vi "启动.vi"() -> ()   [LabVIEW 2016]
uses:
  <vilib>/NI/Progress Bar/Controls/Update Bar Actions.ctl
  <vilib>/NI/Progress Bar/Controls/Progress Bar Properties.ctl
  <vilib>/NI/Progress Bar/Progress Bar.lvlib
panel:
  out "exists?":bool
  out "error out":errorcluster
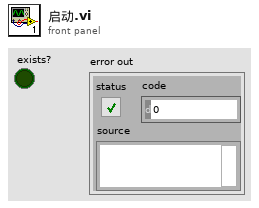
[diagram p1: front panel]
types:
  T1 = enum32{"Invalid", "Standard", "Closed", "Hidden", "Minimized", "Maximized"}
  T2 = typedef "Progress Bar.lvlib/Progress Bar Properties.ctl" = cluster{"Background Color":u32, "Installer Title":string, "Title Color":u32, "Action Text":string, "Text Color":u32, "Slider Value":u8, "Bar Color":u32, "Timeout":i32}
  T3 = typedef "Progress Bar.lvlib/Update Bar Actions.ctl" = enum16{"Add To Existing", "Set to Value"}
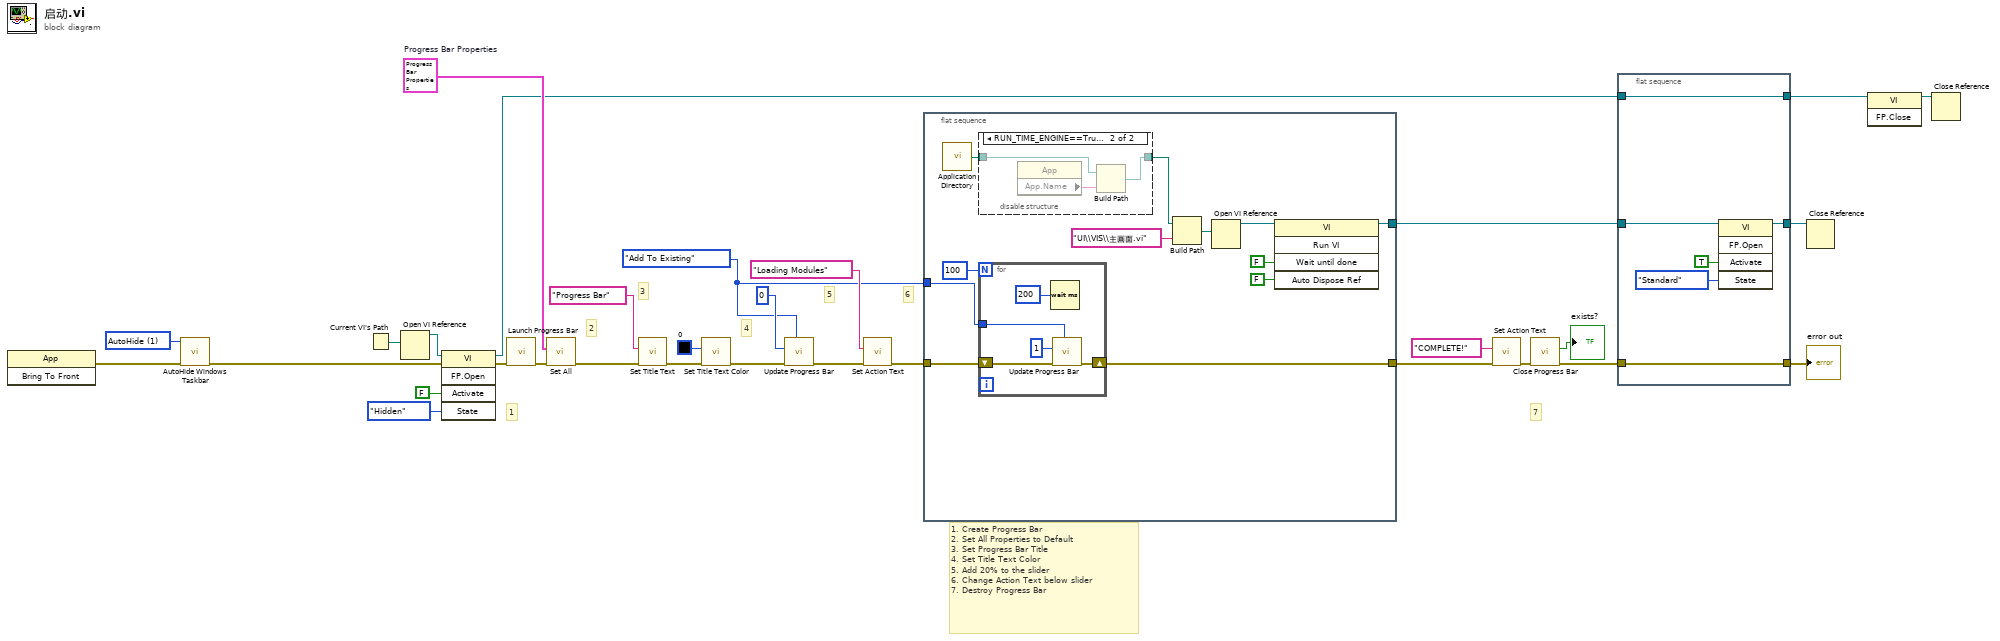
[diagram p0: block diagram]
diagram:
  w4 = u8 1 items=["AutoHide"=1, "AlwaysOnTop"=2] ("Operation")
  w20 = T2 {"Background Color"=3381759, "Installer Title"="Progress", "Title Color"=0, "Action Text"="", "Text Color"=0, "Slider Value"=0, "Bar Color"=6618880, "Timeout"=10000}  # Progress Bar Properties
  w19 = Update_Bar_Actions."Add To Existing" ("Action")
  # "7"
  # "6"
  # "5"
  # "4"
  # "3"
  # "2"
  # "1"
  # "1. Create Progress Bar\n2. Set All Properties to Default\n3. Set Progress Bar Title\n4. Set Title Text Color\n5. Add 20% to the slider\n6. Change Action Text below slider\n7. Destroy Progress Bar"
  n1 = invoke class="App" method="Bring To Front"() -> (error out=w2:errorcluster)  [unwired: 3 in, 2 out]
  n2 = call "AutoHide Windows Taskbar.vi"("error in (no error)"=w2, "Operation"=w4) -> ("error out"=w5:errorcluster)  [unwired: 5 in]
  n3 = Current VI's Path() -> (path=w14:path)
  n4 = Open VI Reference(vi path=w14) -> (vi reference=w15:refnum<vi>)  [unwired: 5 in, 1 out]
  n5 = invoke class="VI" method="FP.Open"(reference=w15, error in=w5, "Activate"=FALSE ("激活？"), "State"=T1."Hidden" ("状态")) -> (reference out=w10:refnum<vi>, error out=w11:errorcluster)  [unwired: 1 in, 3 out]
  n6 = call <vilib>:"Launch Progress Bar.vi"("error in (no error)"=w11) -> ("error out"=w21:errorcluster)  [unwired: 9 in, 1 out]
  n7 = call <vilib>:"Set All.vi"("error in (no error)"=w21, "Progress Bar Properties (Default)"=w20) -> ("error out"=w27:errorcluster)  [unwired: 9 in]
  n8 = call <vilib>:"Set Title Text.vi"("error in (no error)"=w27, "Installer Title"="Progress Bar") -> ("error out"=w30:errorcluster)  [unwired: 9 in]
  n9 = call <vilib>:"Set Title Text Color.vi"("error in (no error)"=w30, "Color Box"=u32 0) -> ("error out"=w26:errorcluster)  [unwired: 9 in]
  n10 = call <vilib>:"Update Progress Bar.vi"("Action"=w19, "error in (no error)"=w26, "Value"=u8 0) -> ("error out"=w1:errorcluster)  [unwired: 8 in]
  n11 = call <vilib>:"Set Action Text.vi"("error in (no error)"=w1, "Action Text"="Loading Modules") -> ("error out"=w24:errorcluster)  [unwired: 9 in]
  n12 = flat-sequence {
    tunnel: w24 -> [w43]
    tunnel: [w42] -> w23
    tunnel: w19 -> [w41]
    tunnel: [w39] -> w9
    frame #0 {
      n13 = call <vilib>:"Application Directory.vi"() -> ("Application Directory"=w38:path)
      n14 = disable-structure shown="RUN_TIME_ENGINE==True" {
        disable-tunnel: w38 -> [w44 w47]
        disable-tunnel: [w44 w45] -> w36
        frame condition #0 (active) {
        }
        frame condition #1 {
          n15 = property class="App"() -> ("App.Name"=w46:string)  [unwired: 2 in, 2 out]
          n16 = Build Path(base path=w47, name or relative path=w46) -> (appended path=w45:path)
        }
      }
      n17 = for {
        N: 100 ("Value") -> [_]
        tunnel: w41 -> [w49]
        shift-right: [w52] -> w42
        shift-left: w43 -> [w51]
        n18 = Wait (ms)(milliseconds to wait=u32 200) -> ()  [unwired: 1 out]
        n19 = call <vilib>:"Update Progress Bar.vi"("Action"=w49, "error in (no error)"=w51, "Value"=u8 1) -> ("error out"=w52:errorcluster)  [unwired: 8 in]
      }
      n20 = Build Path(base path=w36, name or relative path="UI\\VIS\\主画面.vi" ("名称或相对路径")) -> (appended path=w33:path)
      n21 = Open VI Reference(vi path=w33) -> (vi reference=w32:refnum<vi>)  [unwired: 5 in, 1 out]
      n22 = invoke class="VI" method="Run VI"(reference=w32, "Wait until done"=FALSE ("结束前等待"), "Auto Dispose Ref"=FALSE ("自动销毁引用")) -> (reference out=w39:refnum<vi>)  [unwired: 2 in, 4 out]
    }
  }
  n23 = call <vilib>:"Set Action Text.vi"("error in (no error)"=w23, "Action Text"="COMPLETE!") -> ("error out"=w8:errorcluster)  [unwired: 9 in]
  n24 = call <vilib>:"Close Progress Bar.vi"("error in (no error)"=w8) -> ("error out"=w7:errorcluster, "exists?"=→"exists?":bool)  [unwired: 9 in]
  n25 = flat-sequence {
    tunnel: w7 -> [w58]
    tunnel: [w58] -> w6
    tunnel: [w57] -> w16
    tunnel: w10 -> [w57]
    tunnel: w9 -> [w56]
    tunnel: [w55] -> w3
    frame #0 {
      n26 = invoke class="VI" method="FP.Open"(reference=w56, "Activate"=TRUE ("激活？"), "State"=T1."Standard" ("状态")) -> (reference out=w55:refnum<vi>)  [unwired: 2 in, 4 out]
    }
  }
  n27 = Close Reference(reference=w3) -> ()  [unwired: 1 in, 1 out]
  n28 = invoke class="VI" method="FP.Close"(reference=w16) -> (reference out=w17:refnum<vi>)  [unwired: 2 in, 2 out]
  n29 = Close Reference(reference=w17) -> ()  [unwired: 1 in, 1 out]
  "error out" <- w6
